vi "20T_Set_Monitor_Values.vi"(5 "System Monitor Variables (in)":T1) -> (1 "System Monitor Variables (out)":T1)   [LabVIEW 2019]
uses:
  Global/Global Variables/System Monitor Cluster.ctl
  Global/Global Variables/Data_Display_global.vi
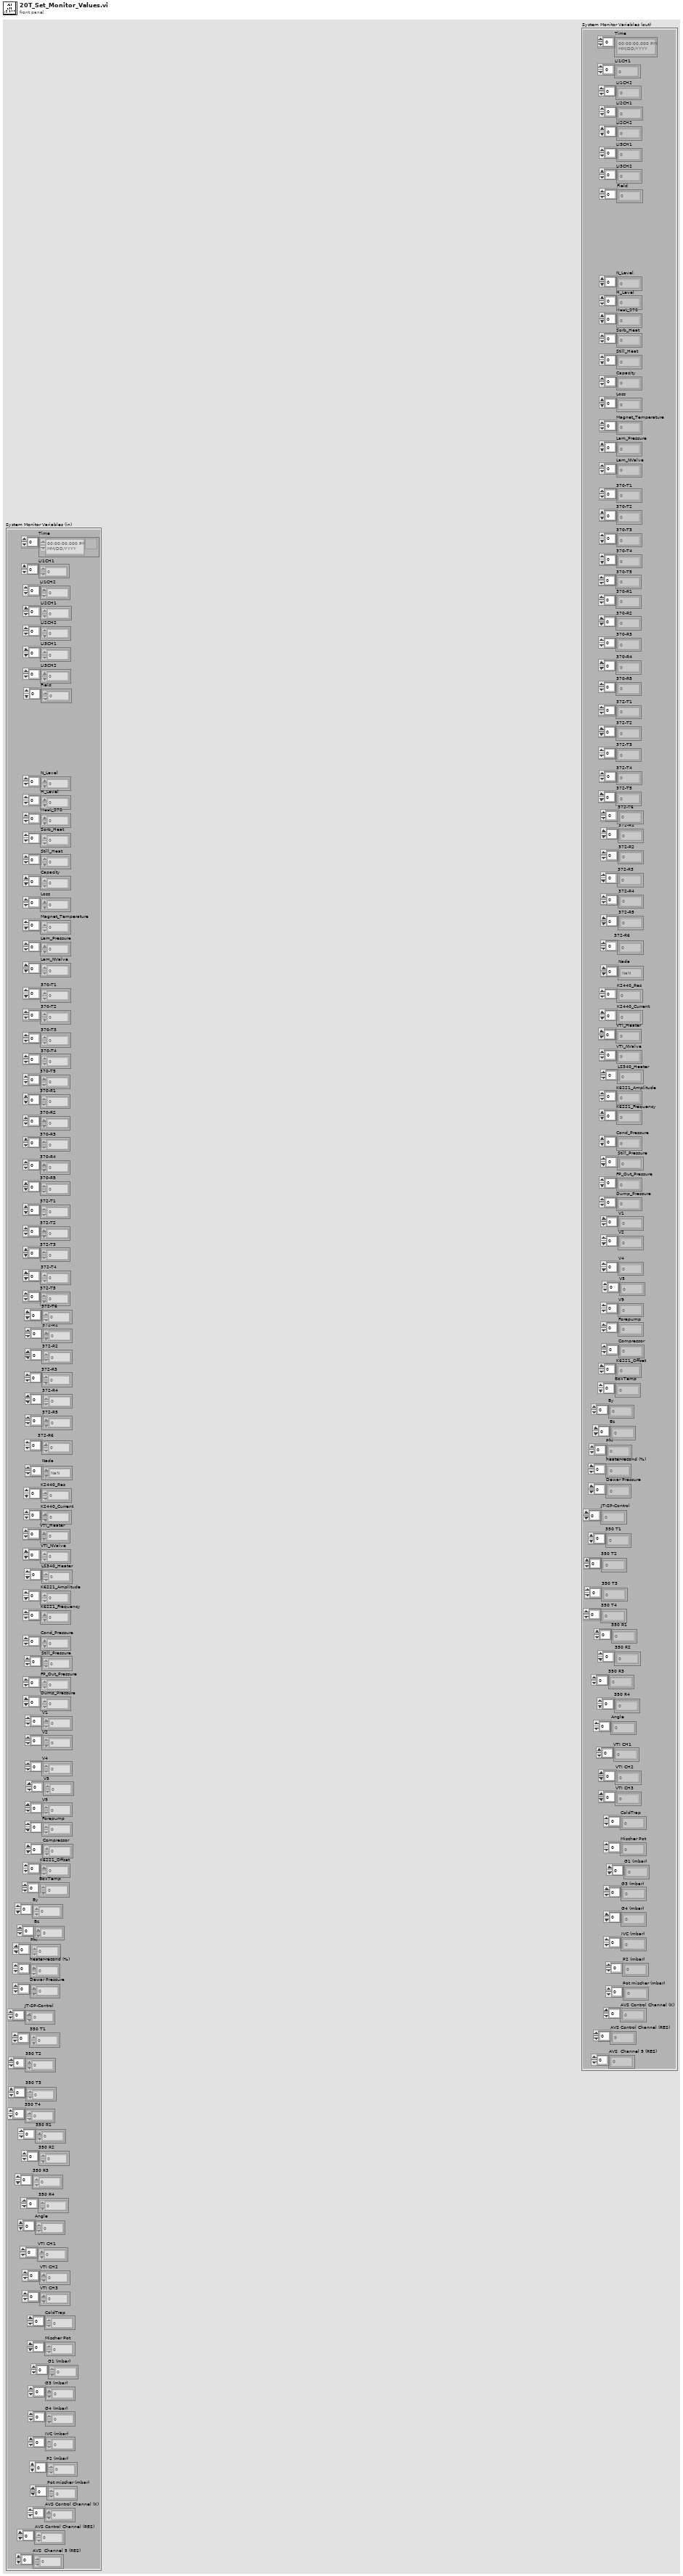
[diagram p1: front panel]
types:
  T1 = typedef "System Monitor Cluster.ctl" = cluster{"Time":timestamp[], "LI1CH1":dbl[], "LI1CH2":dbl[], "LI2CH1":dbl[], "LI2CH2":dbl[], "LI3CH1":dbl[], "LI3CH2":dbl[], "Field":dbl[], "N_Level":dbl[], "H_Level":dbl[], "Heat_370":dbl[], "Sorb_Heat":dbl[], "Still_Heat":dbl[], "Capacity":dbl[], "Loss":dbl[], "Magnet_Temperature":dbl[], "Lam_Pressure":dbl[], "Lam_NValve":dbl[], "370-T1":dbl[], "370-T2":dbl[], "370-T3":dbl[], "370-T4":dbl[], "370-T5":dbl[], "370-R1":dbl[], "370-R2":dbl[], "370-R3":dbl[], "370-R4":dbl[], "370-R5":dbl[], "372-T1":dbl[], "372-T2":dbl[], "372-T3":dbl[], "372-T4":dbl[], "372-T5":dbl[], "372-T6":dbl[], "372-R1":dbl[], "372-R2":dbl[], "372-R3":dbl[], "372-R4":dbl[], "372-R5":dbl[], "372-R6":dbl[], "Nada":dbl[], "K2440_Res":dbl[], "K2440_Current":dbl[], "VTI_Heater":dbl[], "VTI_NValve":dbl[], "LS340_Heater":dbl[], "K6221_Amplitude":dbl[], "K6221_Frequency":dbl[], "Cond_Pressure":dbl[], "Still_Pressure":dbl[], "FP_Out_Pressure":dbl[], "Dump_Pressure":dbl[], "V1":dbl[], "V2":dbl[], "V4":dbl[], "V5":dbl[], "V9":dbl[], "Forepump":dbl[], "Compressor":dbl[], "K6221_Offset":dbl[], "BoxTemp":dbl[], "By":dbl[], "Bz":dbl[], "Phi":dbl[], "heater-recond (%)":dbl[], "Dewar Pressure ":dbl[], "JT-SP-Control":dbl[], "350 T1":dbl[], "350 T2":dbl[], "350 T3":dbl[], "350 T4":dbl[], "350 R1":dbl[], "350 R2":dbl[], "350 R3":dbl[], "350 R4":dbl[], "Angle":dbl[], "VTI CH1":dbl[], "VTI CH2":dbl[], "VTI CH3":dbl[], "ColdTrap":dbl[], "Mischer Pot":dbl[], "G1 (mbar)":dbl[], "G3 (mbar) ":dbl[], "G4 (mbar)":dbl[], "IVC (mbar)":dbl[], "P2 (mbar) ":dbl[], "Pot mischer (mbar)":dbl[], "AVS Control Channel (K)":dbl[], "AVS Control Channel (RES)":dbl[], "AVS  Channel 5 (RES) ":dbl[]}
  T2 = typedef "20T_Cluster.ctl" = cluster{"Clamp":bool, "Switch Heater":bool, "Go to Zero":bool, "Go to set":bool, "Go to Hold":bool, "Clamped":bool, "Quenched":bool, "Rate limit":bool, "Persistent":bool, "Hold":bool, "Set":bool, "Zero":bool, "Magnet (T)":dbl, "Leads (T)":dbl, "Magnet T (K)":dbl, "Switch":bool, "Target (T)":dbl, "Setpoint (T)":dbl, "Rate (T/min)":dbl, "Switch Heater 2":bool, "Set Rate":bool}
  T3 = typedef "20T_Dewar_Cluster.ctl" = cluster{"Dewar Heater (%) Bar":dbl, "Dewar-Heater (%) Display":dbl, "Dewar-Heater (%) SP":dbl, "Set Dewar-Heater SP":bool, "Change D-Heater Status":bool, "Dewar Pressure":dbl, "Dewar heater manual":bool, "Dewar Heater (W)":dbl}
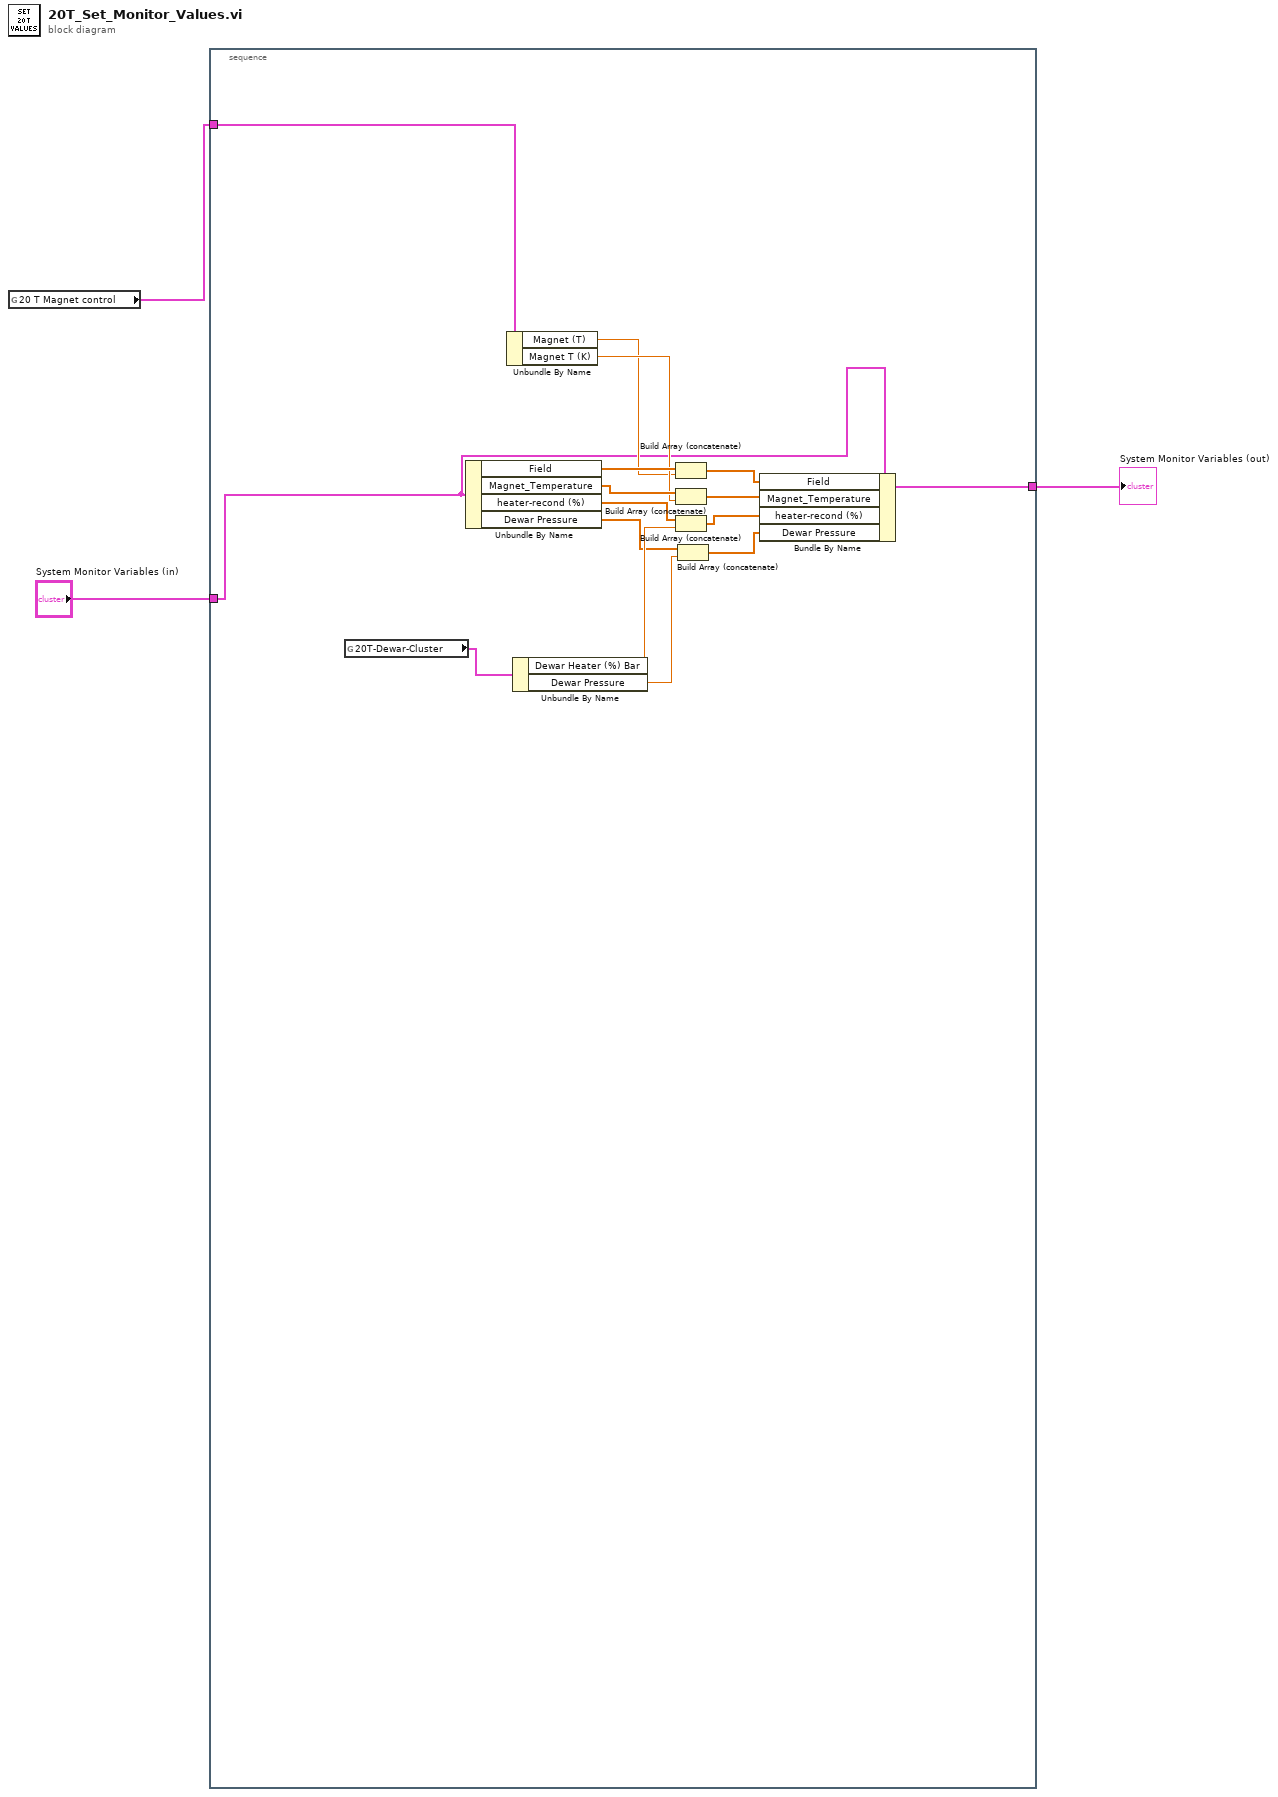
[diagram p0: block diagram]
diagram:
  n1 = global read "Data_Display_global.vi" "20 T Magnet control"() -> (w2:T2)
  n2 = stacked-sequence {
    tunnel: "System Monitor Variables (in)" -> [w11]
    tunnel: w2 -> [w19]
    tunnel: [w14] -> w1
    frame #0 {
      n3 = global read "Data_Display_global.vi" "20T-Dewar-Cluster"() -> (w10:T3)
      n4 = Unbundle By Name(w11) -> ("Field"=w18:dbl[], "Magnet_Temperature"=w17:dbl[], "heater-recond (%)"=w6:dbl[], "Dewar Pressure"=w7:dbl[])
      n5 = Unbundle By Name(w19) -> ("Magnet (T)"=w15:dbl, "Magnet T (K)"=w16:dbl)
      n6 = Unbundle By Name(w10) -> ("Dewar Heater (%) Bar"=w9:dbl, "Dewar Pressure"=w8:dbl)
      n7 = Build Array (concatenate)(w18, w15) -> (w12:dbl[])
      n8 = Build Array (concatenate)(w17, w16) -> (w13:dbl[])
      n9 = Build Array (concatenate)(w6, w9) -> (w5:dbl[])
      n10 = Build Array (concatenate)(w7, w8) -> (w4:dbl[])
      n11 = Bundle By Name(cluster=w11, "Field"=w12, "Magnet_Temperature"=w13, "heater-recond (%)"=w5, "Dewar Pressure"=w4) -> (w14:T1)
    }
  }
  "System Monitor Variables (out)" <- w1
